vi "Debug Board 2D String to 1D Cluster.vi"(0 "Debug Board 2D String":T1=[["", "", "A", "", "A", "AK", "A"], ["", "", "", "", "AK", "AA", "A"], ["", "B", "", "", "", "A", ""], ["B", "B", "B", "B", "", "", ""], ["B", "", "A", "", "A", "", ""], ["B", "", "", "", "", "", "A"], ["", "", "A", "A", "", "", ""]]) -> (4 "1D Board":T2[](array[typedef])=[{"Team"=0, "Occu."=enum."N", "Count"=0}, {"Team"=0, "Occu."=enum."N", "Count"=0}, {"Team"=1, "Occu."=enum."C", "Count"=1}, {"Team"=0, "Occu."=enum."N", "Count"=0}, {"Team"=1, "Occu."=enum."N", "Count"=1}, {"Team"=1, "Occu."=enum."C", "Count"=0}, {"Team"=1, "Occu."=enum."N", "Count"=1}, {"Team"=0, "Occu."=enum."N", "Count"=0}, {"Team"=0, "Occu."=enum."N", "Count"=0}, {"Team"=0, "Occu."=enum."N", "Count"=0}, {"Team"=0, "Occu."=enum."N", "Count"=0}, {"Team"=1, "Occu."=enum."K", "Count"=0}, {"Team"=1, "Occu."=enum."C", "Count"=2}, {"Team"=1, "Occu."=enum."C", "Count"=1}, {"Team"=0, "Occu."=enum."N", "Count"=0}, {"Team"=2, "Occu."=enum."C", "Count"=1}, {"Team"=0, "Occu."=enum."N", "Count"=0}, {"Team"=0, "Occu."=enum."N", "Count"=0}, {"Team"=0, "Occu."=enum."N", "Count"=0}, {"Team"=1, "Occu."=enum."C", "Count"=1}, {"Team"=0, "Occu."=enum."N", "Count"=0}, {"Team"=2, "Occu."=enum."C", "Count"=1}, {"Team"=2, "Occu."=enum."C", "Count"=1}, {"Team"=2, "Occu."=enum."C", "Count"=1}, {"Team"=2, "Occu."=enum."C", "Count"=1}, {"Team"=0, "Occu."=enum."N", "Count"=0}, {"Team"=0, "Occu."=enum."N", "Count"=0}, {"Team"=0, "Occu."=enum."N", "Count"=0}, {"Team"=2, "Occu."=enum."C", "Count"=1}, {"Team"=0, "Occu."=enum."N", "Count"=0}, {"Team"=1, "Occu."=enum."C", "Count"=1}, {"Team"=0, "Occu."=enum."N", "Count"=0}, {"Team"=1, "Occu."=enum."C", "Count"=1}, {"Team"=0, "Occu."=enum."N", "Count"=0}, {"Team"=0, "Occu."=enum."N", "Count"=0}, {"Team"=2, "Occu."=enum."C", "Count"=1}, {"Team"=0, "Occu."=enum."N", "Count"=0}, {"Team"=0, "Occu."=enum."N", "Count"=0}, {"Team"=0, "Occu."=enum."N", "Count"=0}, {"Team"=0, "Occu."=enum."N", "Count"=0}, {"Team"=0, "Occu."=enum."N", "Count"=0}, {"Team"=1, "Occu."=enum."C", "Count"=1}, {"Team"=0, "Occu."=enum."N", "Count"=0}, {"Team"=0, "Occu."=enum."N", "Count"=0}, {"Team"=1, "Occu."=enum."C", "Count"=1}, {"Team"=1, "Occu."=enum."C", "Count"=1}, {"Team"=0, "Occu."=enum."N", "Count"=0}, {"Team"=0, "Occu."=enum."N", "Count"=0}, {"Team"=0, "Occu."=enum."N", "Count"=0}])   [LabVIEW 2014, in "Dragon Tamers.lvlib"]
uses:
  Dragon Tamers.lvlib
  Typedefs/Board Cell.ctl
  Typedefs/Cell Occupancy.ctl
  Typedefs/Debug Board 2D String.ctl
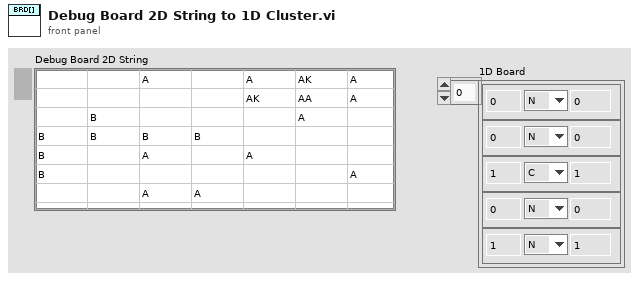
[diagram p1: front panel]
types:
  T1 = typedef "Dragon Tamers.lvlib/Debug Board 2D String.ctl" = string[][]
  T2 = typedef "Dragon Tamers.lvlib/Board Cell.ctl" = cluster{"Team":i32, "Occu.":T3, "Count":i32}
  T3 = typedef "Dragon Tamers.lvlib/Cell Occupancy.ctl" = enum16{"N", "C", "K"}
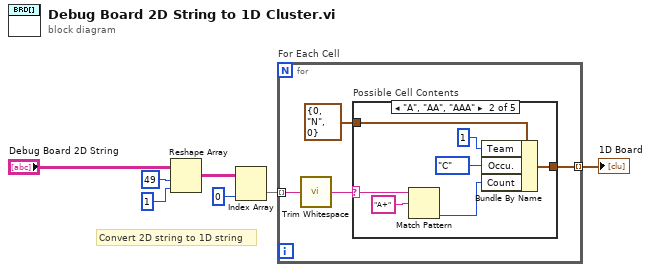
[diagram p0: block diagram]
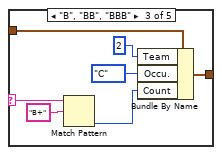
[diagram p3: hidden frame]
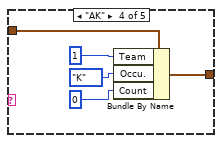
[diagram p4: hidden frame]
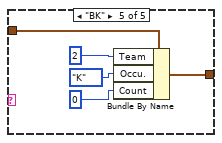
[diagram p5: hidden frame]
diagram:
  # "Convert 2D string to 1D string"
  n1 = Reshape Array("Debug Board 2D String", 49 ("dimension size"), 1 ("dimension size")) -> (w4:T1)
  n2 = Index Array(array=w4, index (col)=0 ("disabled index (col)")) -> (element=w2:string[])  [unwired: 1 in]
  n3 = for "For Each Cell" {
    tunnel: w2 -> [w11] mode=indexing
    tunnel: [w9] -> w1 mode=indexing
    n4 = call <vilib>:"Trim Whitespace.vi"("string"=w11) -> ("trimmed string"=w8:string)  [unwired: 1 in]
    n5 = case "Possible Cell Contents" shown="\"A\", \"AA\", \"AAA\"" w8 {
      selector: w8 -> [_ w19 w26 _ _]
      tunnel: T2 {"Team"=0, "Occu."=enum."N", "Count"=0} ("Cell") -> [w12 w17 w24 w31 w36]
      tunnel: [w12 w13 w20 w28 w33] -> w9
      frame Default {
      }
      frame "A", "AA", "AAA" {
        n6 = Match Pattern(string=w19, regular expression="A+") -> (offset past match=w14:i32)  [unwired: 1 in, 3 out]
        n7 = Bundle By Name(cluster=w17, "Team"=1, "Occu."=Cell_Occupancy."C", "Count"=w14) -> (w13:T2)
      }
      frame "B", "BB", "BBB" {
        n8 = Match Pattern(string=w26, regular expression="B+") -> (offset past match=w21:i32)  [unwired: 1 in, 3 out]
        n9 = Bundle By Name(cluster=w24, "Team"=2, "Occu."=Cell_Occupancy."C", "Count"=w21) -> (w20:T2)
      }
      frame "AK" {
        n10 = Bundle By Name(cluster=w31, "Team"=1, "Occu."=Cell_Occupancy."K", "Count"=0) -> (w28:T2)
      }
      frame "BK" {
        n11 = Bundle By Name(cluster=w36, "Team"=2, "Occu."=Cell_Occupancy."K", "Count"=0) -> (w33:T2)
      }
    }
  }
  "1D Board" <- w1
